vi "Start Triggers Sync AUX.vi"(0 "sync.resources":T8, 5 "rx.parameters":T7={"rx.trigger select"=enum."Software", "rx.trigger enable"=FALSE, "rx.trigger sync enable"=FALSE, "rx 0.stream enable"=FALSE, "rx 1.stream enable"=FALSE, "rx.software trigger"=FALSE, "rx.reset"=FALSE, "rx.abort"=FALSE, "rx.samples to acquire"=0, "ddc parameters"=[{"output sample rate"=0.0, "delay"=0.0, "frequency shift"=0.0, "impairments"={"inline gain I"=0.0, "inline gain Q"=0.0, "cross gain I"=0.0, "cross gain Q"=0.0, "pre-gain offset I"=0.0, "pre-gain offset Q"=0.0, "post-gain offset I"=0.0, "post-gain offset Q"=0.0}, "phase"=0.0}, {"output sample rate"=0.0, "delay"=0.0, "frequency shift"=0.0, "impairments"={"inline gain I"=0.0, "inline gain Q"=0.0, "cross gain I"=0.0, "cross gain Q"=0.0, "pre-gain offset I"=0.0, "pre-gain offset Q"=0.0, "post-gain offset I"=0.0, "post-gain offset Q"=0.0}, "phase"=0.0}]} {"ddc parameters"."frequency shift" format="%#.48g"}, 7 "tx.parameters":T5={"tx.trigger select"=enum."Software", "tx.trigger enable"=FALSE, "tx.trigger sync enable"=FALSE, "tx 0.stream enable"=FALSE, "tx 1.stream enable"=FALSE, "tx.software trigger"=FALSE, "tx.reset"=FALSE, "tx.abort"=FALSE, "tx.samples to generate"=0, "duc parameters"=[{"frequency shift"=0.0, "impairments"={"inline gain I"=0.0, "inline gain Q"=0.0, "cross gain I"=0.0, "cross gain Q"=0.0, "pre-gain offset I"=0.0, "pre-gain offset Q"=0.0, "post-gain offset I"=0.0, "post-gain offset Q"=0.0}, "phase"=0.0, "input sample rate"=0.0, "gain"={"gain I"=0.0, "gain Q"=0.0}, "delay"=0.0}, {"frequency shift"=0.0, "impairments"={"inline gain I"=0.0, "inline gain Q"=0.0, "cross gain I"=0.0, "cross gain Q"=0.0, "pre-gain offset I"=0.0, "pre-gain offset Q"=0.0, "post-gain offset I"=0.0, "post-gain offset Q"=0.0}, "phase"=0.0, "input sample rate"=0.0, "gain"={"gain I"=0.0, "gain Q"=0.0}, "delay"=0.0}]} {"duc parameters"."frequency shift" format="%#.48g"}) -> (4 "rx.start trigger":bool, 6 "tx.start trigger":bool)   [LabVIEW 2023]
uses:
  <instrlib>/niUSRPRIO/Synchronization/v1/FPGA/Private/Resources.ctl
  <instrlib>/niUSRPRIO/Synchronization/v1/FPGA/niUsrpRio Synchronization v1 FPGA.lvlib
  <instrlib>/_niInstr/DSP/v1/Shared/Public/IQ Impairments.ctl
  <instrlib>/niUSRP/Reference FPGA/SubVIs/DDC Parameters.ctl
  <instrlib>/niVST/Reference FPGA/FPGA/USRPRIO Sample VIs/Host/SubVIs/Start Trigger.ctl
  <instrlib>/_niInstr/DSP/v1/Shared/Public/IQ Gain.ctl
  <instrlib>/niUSRP/Reference FPGA/SubVIs/DUC Parameters.ctl
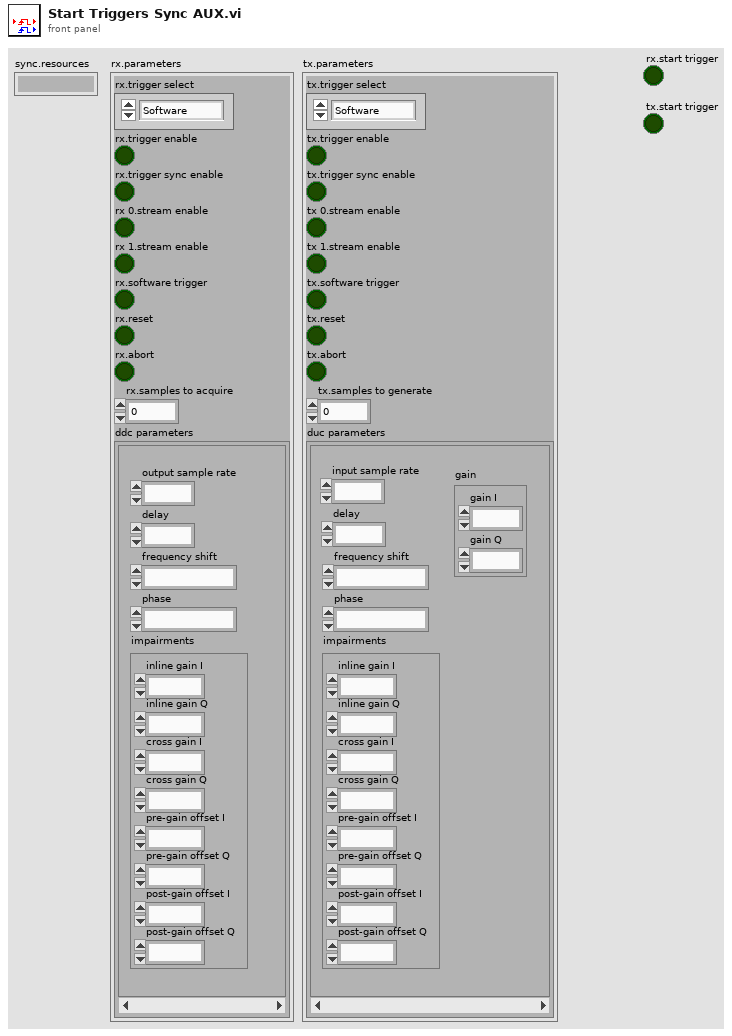
[diagram p1: front panel]
types:
  T1 = typedef "Start Trigger.ctl" = enum8{"Software", "Digital Edge", "Rx Start Trigger", "Tx Start Trigger", "Immediate", "Future Time Event"}
  T2 = typedef "DUC Parameters.ctl" = cluster{"frequency shift":fxp<+/-,48,0>, "impairments":T3, "phase":fxp<+/-,21,0>, "input sample rate":fxp<+,48,1>, "gain":T4, "delay":fxp<+/-,18,0>}
  T3 = typedef "niInstr DSP v1 Shared.lvlib/IQ Impairments.ctl" = cluster{"inline gain I":fxp<+/-,18,1>, "inline gain Q":fxp<+/-,18,1>, "cross gain I":fxp<+/-,18,1>, "cross gain Q":fxp<+/-,18,1>, "pre-gain offset I":fxp<+/-,18,1>, "pre-gain offset Q":fxp<+/-,18,1>, "post-gain offset I":fxp<+/-,18,1>, "post-gain offset Q":fxp<+/-,18,1>}
  T4 = typedef "niInstr DSP v1 Shared.lvlib/IQ Gain.ctl" = cluster{"gain I":fxp<+/-,24,3>, "gain Q":fxp<+/-,24,3>}
  T5 = cluster{"tx.trigger select":T1, "tx.trigger enable":bool, "tx.trigger sync enable":bool, "tx 0.stream enable":bool, "tx 1.stream enable":bool, "tx.software trigger":bool, "tx.reset":bool, "tx.abort":bool, "tx.samples to generate":u32, "duc parameters":T2[]}
  T6 = typedef "DDC Parameters.ctl" = cluster{"output sample rate":fxp<+,48,1>, "delay":fxp<+/-,16,0>, "frequency shift":fxp<+/-,48,0>, "impairments":T3, "phase":fxp<+/-,21,0>}
  T7 = cluster{"rx.trigger select":T1, "rx.trigger enable":bool, "rx.trigger sync enable":bool, "rx 0.stream enable":bool, "rx 1.stream enable":bool, "rx.software trigger":bool, "rx.reset":bool, "rx.abort":bool, "rx.samples to acquire":u32, "ddc parameters":T6[]}
  T8 = typedef "niUsrpRio Synchronization v1 FPGA.lvlib/Resources.ctl" = cluster{"master":refnum<k21>, "meas.enable":refnum<k21>, "meas.ready":refnum<k21>, "meas.reset":refnum<k21>, "meas.arm":refnum<k21>, "meas.valid":refnum<k21>, "meas.value":refnum<k21>, "meas.oversample factor":refnum<k21>, "cptr":refnum<k21>, "cptr.adjust":refnum<k21>, "cptr.period":refnum<k21>}
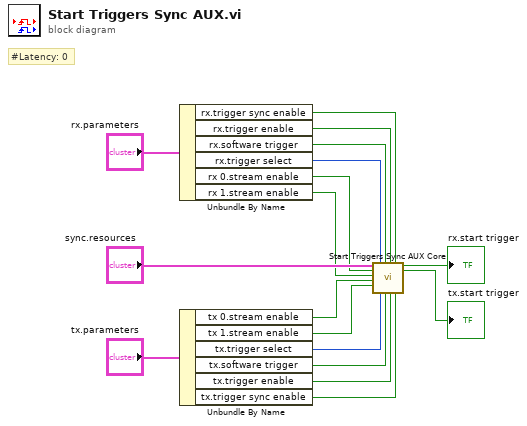
[diagram p0: block diagram]
diagram:
  # "#Latency: 0"
  n1 = Unbundle By Name("rx.parameters") -> ("rx.trigger sync enable"=w15:bool, "rx.trigger enable"=w14:bool, "rx.software trigger"=w13:bool, "rx.trigger select"=w12:T1, "rx 0.stream enable"=w11:bool, "rx 1.stream enable"=w10:bool)
  n2 = Unbundle By Name("tx.parameters") -> ("tx 0.stream enable"=w8:bool, "tx 1.stream enable"=w7:bool, "tx.trigger select"=w6:T1, "tx.software trigger"=w5:bool, "tx.trigger enable"=w4:bool, "tx.trigger sync enable"=w3:bool)
  n3 = call <instrlib>:"Start Triggers Sync AUX Core.vi"("sync.resources"="sync.resources", "rx 0.stream enable"=w11, "rx 1.stream enable"=w10, "tx 0.stream enable"=w8, "tx 1.stream enable"=w7, "rx.trigger select"=w12, "tx.trigger select"=w6, "rx.software trigger"=w13, "tx.software trigger"=w5, "rx.trigger enable"=w14, "tx.trigger enable"=w4, "rx.trigger sync enable"=w15, "tx.trigger sync enable"=w3) -> ("rx.start trigger"=→"rx.start trigger":bool, "tx.start trigger"=→"tx.start trigger":bool)  [unwired: 5 in]
